vi "Handle Errors.vi"(8 "error in (no error)":errorcluster) -> (0 "error out":errorcluster)   [LabVIEW 2020, in "Process.lvclass"]
uses:
  Process.lvclass
  Support/Utilities.lvlib
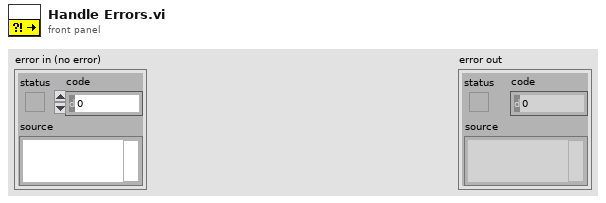
[diagram p1: front panel]
types:
  T1 = enum16{"open", "replace", "create", "open or create", "replace or create", "replace or create with confirmation"}
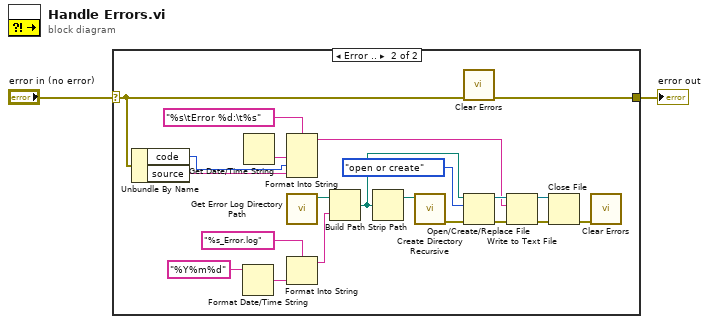
[diagram p0: block diagram]
diagram:
  n1 = case shown="Error .." "error in (no error)" {
    selector: "error in (no error)" -> [w3 w23]
    tunnel: [w3 w24] -> w1
    frame No Error {
    }
    frame Error {
      n2 = Unbundle By Name(w23) -> ("code"=w7:i32, "source"=w6:string)
      n3 = Format Date/Time String(time format string (%c)="%Y%m%d") -> (date/time string=w22:string)  [unwired: 2 in]
      n4 = Get Date/Time String() -> (time string=w5:string)  [unwired: 3 in, 1 out]
      n5 = Format Into String(format string="%s\tError %d:\t%s", w5, w7, w6) -> (resulting string=w4:string)  [unwired: 2 in, 1 out]
      n6 = call "Get Error Log Directory Path.vi"() -> ("Error Log Path"=w16:path)  [unwired: 11 in]
      n7 = Format Into String(format string="%s_Error.log", w22) -> (resulting string=w15:string)  [unwired: 2 in, 1 out]
      n8 = Build Path(base path=w16, name or relative path=w15) -> (appended path=w14:path)
      n9 = Strip Path(path=w14) -> (stripped path=w19:path)  [unwired: 1 out]
      n10 = call <vilib>:"Create Directory Recursive.vi"("directory"=w19) -> ("error out"=w20:errorcluster)  [unwired: 4 in, 2 out]
      n11 = call <vilib>:"Clear Errors.vi"("error in (no error)"=w23) -> ("error out"=w24:errorcluster)  [unwired: 5 in, 1 out]
      n12 = Open/Create/Replace File(file path (use dialog)=w14, error in=w20, operation (0:open)=T1."open or create") -> (refnum out=w13:refnum<file>, error out=w12:errorcluster)  [unwired: 3 in, 1 out]
      n13 = Write to Text File(file (use dialog)=w13, text=w4, error in=w12) -> (refnum out=w11:refnum<file>, error out=w10:errorcluster)  [unwired: 1 in, 1 out]
      n14 = Close File(refnum=w11, error in=w10) -> (error out=w9:errorcluster)  [unwired: 1 out]
      n15 = call <vilib>:"Clear Errors.vi"("error in (no error)"=w9) -> ()  [unwired: 5 in, 2 out]
    }
  }
  "error out" <- w1
